vi "user process.vi"(8 "error in":errorcluster, 11 "Parameters to process":T2) -> (0 "error out":errorcluster, 3 "Results from processing":T1)   [LabVIEW 2013, in "user control module.lvclass"]
uses:
  user control module.lvclass
  scripting/FixedChannelTBModuleDecideFeatures.lvclass
  result user data.ctl
  parameter user data.ctl
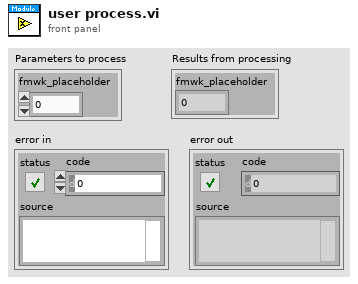
[diagram p1: front panel]
types:
  T1 = typedef "user control module.lvclass/result user data.ctl" = cluster{"fmwk_placeholder":sgl}
  T2 = typedef "user control module.lvclass/parameter user data.ctl" = cluster{"fmwk_placeholder":sgl}
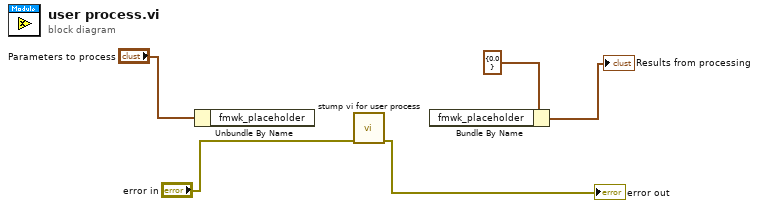
[diagram p0: block diagram]
diagram:
  n1 = Unbundle By Name ("Unbundle Parameters to process")("Parameters to process") -> ()  [unwired: 1 out]
  n2 = call "stump vi for user process.vi"("error in (no error)"="error in") -> ("error out"=→"error out":errorcluster)  [unwired: 10 in]
  n3 = Bundle By Name ("Bundle Results from processing")(cluster=T1 {"fmwk_placeholder"=0.0} ("Results from processing")) -> (→"Results from processing":T1)  [unwired: 1 in]
